vi "SetRangeQDC.vi"(7 "Low Range threshold":u16, 8 "error in (no error)":errorcluster, 9 "High range threshold":u16, 10 "handle":i32, 11 "VME module Base Address":u32) -> (0 "error out":errorcluster)   [LabVIEW 2014]
uses:
  Program Files (x86)/CAEN/Comm/labview/CAENComm.lvlib
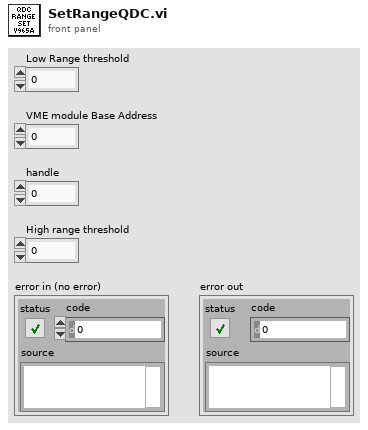
[diagram p1: front panel]
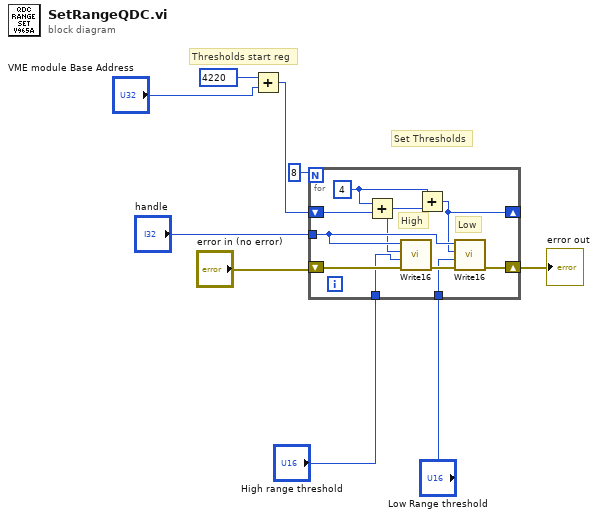
[diagram p0: block diagram]
diagram:
  # "Set Thresholds"
  # "Thresholds start reg"
  n1 = Add(x=u32 4220, y="VME module Base Address") -> (x+y=w7:u32)
  n2 = for {
    N: 8 -> [_]
    shift-right: [w17] -> w4
    shift-left: "error in (no error)" -> [w19]
    tunnel: "handle" -> [w16]
    shift-right: [w12] -> _
    shift-left: w7 -> [w15]
    tunnel: "High range threshold" -> [w11]
    tunnel: "Low Range threshold" -> [w10]
    w13 = u32 4 ("x")
    # "Low"
    # "High"
    n3 = Add(x=w13, y=w15) -> (x+y=w14:u32)
    n4 = call "Write16.vi"("error in (no error)"=w19, "Data"=w11, "Address"=w14, "handle"=w16) -> ("error out"=w18:errorcluster)  [unwired: 7 in]
    n5 = Add(x=w13, y=w14) -> (x+y=w12:u32)
    n6 = call "Write16.vi"("error in (no error)"=w18, "Data"=w10, "Address"=w12, "handle"=w16) -> ("error out"=w17:errorcluster)  [unwired: 7 in]
  }
  "error out" <- w4
